vi "Asynchronous Call Test.vi"   [LabVIEW 2015]
uses:
  source/library/Scripting.lvlib
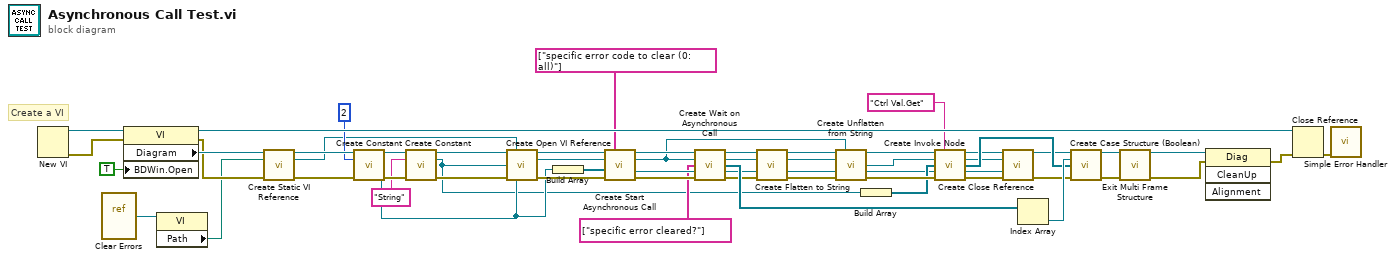
[diagram p0: block diagram]
diagram:
  # "Create a VI"
  n1 = New VI() -> (0:w54:errorcluster, 3:w55:refnum<vi>)  [unwired: 7 in]
  n2 = vi-ref <vilib>:"Clear Errors.vi"() -> (w8:refnum<vi>)
  n3 = property class="VI"(reference=w55, error in=w54, "BDWin.Open"=TRUE ("Block Diagram Window:Open")) -> (reference out=w52:refnum<vi>, error out=w51:errorcluster, "Diagram"=w53:refnum<vi>)
  n4 = property class="VI"(reference=w8) -> ("Path"=w7:path)  [unwired: 1 in, 2 out]
  n5 = call "Create Static VI Reference.vi"("Diagram in"=w53, "VI Path"=w7, "error in (no error)"=w51) -> ("Diagram out"=w47:refnum<vi>, "Terminal"=w32:refnum<vi>, "error out"=w50:errorcluster)  [unwired: 10 in]
  n6 = call "Create Constant.vi"("Diagram in"=w47, "Type"=2, "error in (no error)"=w50) -> ("Diagram out"=w6:refnum<vi>, "Terminal"=w31:refnum<vi>, "error out"=w5:errorcluster)  [unwired: 10 in]
  n7 = call "Create Constant.vi"("Diagram in"=w6, "Type"="String" ("VI Name"), "error in (no error)"=w5) -> ("Diagram out"=w4:refnum<vi>, "Terminal"=w2:refnum<vi>, "error out"=w3:errorcluster)  [unwired: 10 in]
  n8 = call "Create Open VI Reference.vi"("Diagram in"=w4, "type specifier"=w32, "vi path"=w2, "error in (no error)"=w3, "options"=w31) -> ("Diagram out"=w33:refnum<vi>, "vi reference"=w30:refnum<vi>, "error out"=w34:errorcluster)  [unwired: 7 in, 1 out]
  n9 = Build Array(w31) -> (w45:refnum<vi>[])
  n10 = call "Create Start Asynchronous Call.vi"("Diagram in"=w33, "Input Names"=string[] ["specific error code to clear (0: all)"], "reference"=w30, "Inputs"=w45, "error in (no error)"=w34) -> ("Diagram out"=w44:refnum<vi>, "reference out"=w23:refnum<vi>, 10:"error out"=w43:refnum<vi>, 15:"error out"=w49:errorcluster)  [unwired: 7 in]
  n11 = call "Create Wait on Asynchronous Call.vi"("Diagram in"=w44, "reference"=w23, "Output Names"=string[] ["specific error cleared?"], "error in"=w43, "error in (no error)"=w49) -> ("Diagram out"=w28:refnum<vi>, "reference out"=w27:refnum<vi>, "Outputs"=w41:refnum<vi>[], 10:"error out"=w9:refnum<vi>, 15:"error out"=w37:errorcluster)  [unwired: 6 in]
  n12 = call "Create Flatten to String.vi"("Diagram in"=w28, "anything"=w27, "error in"=w9, "error in (no error)"=w37) -> ("Diagram out"=w25:refnum<vi>, "data string"=w24:refnum<vi>, 10:"error out"=w10:refnum<vi>, 15:"error out"=w29:errorcluster)  [unwired: 8 in]
  n13 = call "Create Unflatten from String.vi"("Diagram in"=w25, "type"=w23, "binary string"=w24, "error in"=w10, "error in (no error)"=w29) -> ("Diagram out"=w21:refnum<vi>, "value"=w20:refnum<vi>, 10:"error out"=w11:refnum<vi>, 15:"error out"=w26:errorcluster)  [unwired: 6 in, 1 out]
  n14 = Build Array(w2) -> (w18:refnum<vi>[])
  n15 = call "Create Invoke Node.vi"("Diagram in"=w21, "ID String"="Ctrl Val.Get", "reference"=w20, "Inputs"=w18, "error in"=w11, "error in (no error)"=w26) -> ("Diagram out"=w15:refnum<vi>, "reference out"=w13:refnum<vi>, "Outputs"=w17:refnum<vi>[], 10:"error out"=w12:refnum<vi>, 15:"error out"=w22:errorcluster)  [unwired: 5 in]
  n16 = call "Create Close Reference.vi"("Diagram in"=w15, "application reference"=w13, "error in"=w12, "error in (no error)"=w22) -> ("Diagram out"=w14:refnum<vi>, "error out"=w16:errorcluster)  [unwired: 9 in, 1 out]
  n17 = Index Array(array=w41) -> (element=w38:refnum<vi>)  [unwired: 1 in]
  n18 = call "Create Case Structure (Boolean).vi"("Diagram in"=w14, "Selector"=w38, "Inputs"=w17, "error in (no error)"=w16) -> ("Selected Diagram"=w35:refnum<vi>, "error out"=w36:errorcluster)  [unwired: 8 in, 2 out]
  n19 = call "Exit Multi Frame Structure.vi"("Diagram in"=w35, "error in (no error)"=w36) -> ("Diagram out"=w39:refnum<vi>, "error out"=w40:errorcluster)  [unwired: 11 in, 1 out]
  n20 = invoke class="Diag" method="CleanUp"(reference=w39, error in=w40) -> (error out=w57:errorcluster)  [unwired: 2 in, 3 out]
  n21 = Close Reference(reference=w52, error in (no error)=w57) -> (error out=w56:errorcluster)
  n22 = call <vilib>:"Simple Error Handler.vi"("error in (no error)"=w56) -> ()  [unwired: 4 in, 5 out]
